vi "SPI Flash Read ID.vi"(9 "pID":u8[](array[numeric])=[0, 0, 0, 0, 0, 0, 0, 0, 0, 0, 0, 0, 0, 0, 0, 0, 0, 0, 0, 0, 0, 0, 0, 0, 0, 0, 0, 0, 0, 0, 0, 0], 10 "SPIIndex":i32, 11 "DevHandle":i32) -> (1 "pID out":u8[](array[numeric]), 3 "function return":i32)   [LabVIEW 2010, in "usb2spi.lvlib"]
doc: "int WINAPI SPI_FlashReadID(int DevHandle,int SPIIndex,unsigned char *pID);"
uses:
  usb2spi.lvlib
  USB2XXX/trunk/USB2XXX/USB2XXX/vs2010/Release/USB2XXX.dll
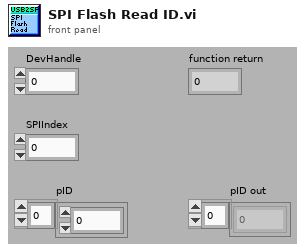
[diagram p1: front panel]
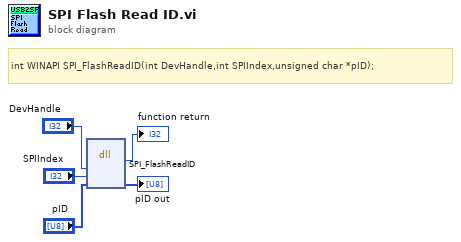
[diagram p0: block diagram]
diagram:
  # "int WINAPI SPI_FlashReadID(int DevHandle,int SPIIndex,unsigned char *pID);"
  n1 = dll-call lib="E:/OtherWork/STM32/USB2XXX/trunk/USB2XXX/USB2XXX/vs2010/Release/USB2XXX.*" fn="SPI_FlashReadID"("DevHandle"="DevHandle", "SPIIndex"="SPIIndex", "pID"="pID") -> (→"function return":i32, "pID"=→"pID out":u8[])  [unwired: 5 in, 2 out]
